vi "Append Front Panel Image.vi"(0 "PDF Report IN":T24(xcontrol), 1 "Scale (%)":sgl=100.0, 3 "Border":T1={"Show?"=FALSE, "Thickness (point)"=0.5, "Color"=0}, 5 "VI reference":refnum<vi>, 9 "visible area only? (T)":bool=TRUE, 11 "error in (no error)":errorcluster, 12 "Caption":string, 14 "Position and indentation":T2={"Alignment"=enum."Center", "X "=0.0, "Y"=0.0, "Indentation"=0.0}) -> (4 "PDF Report OUT":T24(xcontrol), 15 "error out":errorcluster)   [LabVIEW 2012]
doc: "Creates an image of the front panel of the VI you specify in <B>VI reference</B> and appends it to a PDF report.\n\n<B>FRANÇAIS</B>\nCréation de l'image du panneau avant spécifié par <B>VI reference</B> et ajout au rapport PDF.\n\nVersion 1.0\nDeveloped by Jean-Marc Simard\nCopyright © 2010, Exaprom Inc.\nAll rights reserved.\nLicense: BSD\n\nWith iTextSharp 4.1.6 (http://itextsharp.sourceforge.net)\nunder Mozilla Public License Version 1.1\n(http://www.mozilla.org/MPL/MPL-1.1.html)"
uses:
  C:/Users/MaxCorp/Documents/GitHub/TopView/DLL/itextsharp.dll
  GitHub/TopView/DLL/itextsharp.dll
  Controls/Image aligment.ctl
  Controls/Image border.ctl
  Controls/PDF Report Xcontrol/PDF Report.xctl
  Controls/Image alignment and position.ctl
panel:
  out "Size (points)":cluster{"TotalHeight":sgl, "TotalWidth":sgl}
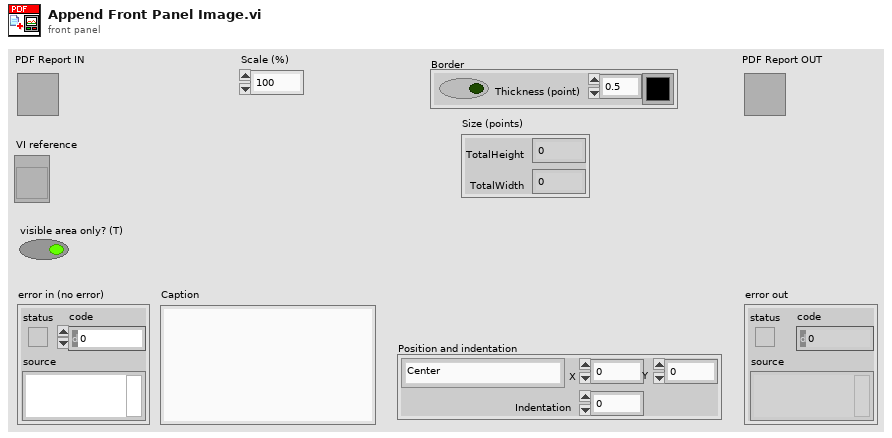
[diagram p1: front panel]
types:
  T1 = typedef "Image border.ctl" = cluster{"Show?":bool, "Thickness (point)":sgl, "Color":u32}
  T2 = typedef "Image alignment and position.ctl" = cluster{"Alignment":T3, "X ":sgl, "Y":sgl, "Indentation":sgl}
  T3 = typedef "Image aligment.ctl" = enum16{"Absolute (X,Y) in mm", "Left", "Center", "Right", "Left (textwrap)", "Right (textwrap)"}
  T4 = typedef "Font cluster.ctl" = cluster{"Name":string, "Size":T5, "Color":T6, "Style":cluster{"Bold":bool, "Italic":bool, "Underline":bool, "Strikeout":bool}}
  T5 = typedef "Font size.ctl" = sgl
  T6 = typedef "Font color.ctl" = u32
  T7 = typedef "Unit.ctl" = enum16{"inch", "mm"}
  T8 = typedef "Paragraphe cluster.ctl" = cluster{" Aligment":T9, "Line spacing":T10}
  T9 = typedef "Texte alignement.ctl" = enum16{"Select", "CENTER", "JUSTIFY", "LEFT", "RIGHT"}
  T10 = typedef "Line spacing.ctl" = enum16{"Select", "1.0", "1.5", "2.0"}
  T11 = typedef "Page dimensions.ctl" = cluster{"Start at page":i32, "Orientation":T12, "widht":sgl, "height":sgl, "Margin left":sgl, "Margin right":sgl, "Margin top":sgl, "Margin bottom":sgl}
  T12 = typedef "Page Orientation.ctl" = enum16{"Portrait", "Landscape"}
  T13 = typedef "Image or Table Caption.ctl" = cluster{"Caption":string, "Separator":string, "Position":enum16{"Above", "Below"}}
  T14 = typedef "Header Footer [ ].ctl" = T15[]
  T15 = typedef "Header Footer cluster.ctl" = cluster{"Start page":i32, "Type":T16, "Alignment":T17, "Vertical Alignement":T18, "Image (%)":sgl, "Page #":T19, "Text":string, "Path":string, "Font":T4, "Font refnum":refnum<k24>, "Line":cluster{"Line":T20, "Thickness (points)":sgl, "Colour":T6}}
  T16 = typedef "Header Footer Type.ctl" = enum16{"Select", "Text", "Text + hyperlink", "Page number", "Image", "Image + hyperlink"}
  T17 = typedef "Header footer horiz alignment.ctl" = enum16{"Left", "Center", "Right"}
  T18 = typedef "Cell Vertical alignment.ctl" = enum16{"TOP", "MIDDLE", "BOTTOM"}
  T19 = typedef "Page number.ctl" = cluster{"Text 1":string, "Text 2":string, "Text 3":string}
  T20 = typedef "Header Footer Line.ctl" = enum16{"No line", "Horizontal line"}
  T21 = typedef "Watermark cluster2.ctl" = cluster{"Show? (F)":bool, "Type":enum16{"Image", "Text"}, "Opacity (%)":sgl, "Rotate(°)":sgl, "Position":cluster{"Position":T22, "X":sgl, "Y":sgl}, "Image path":path, "Scaled(%)":sgl, "Image refnum":refnum<k24>, "Text":string, "Font":cluster{"Name":string, "Size":T5, "Color":T6}, "Font refnum":refnum<k24>, "Alignment":T17, "Automatic":bool}
  T22 = typedef "Watermark Position.ctl" = enum16{"Absolute", "Center (page)", "Center (text section)"}
  T23 = typedef "System Fonts.ctl" = cluster{"Font name [ ]":string[], "Font and file names [ ]":cluster{"Font name":string, "File name":string}[]}
  T24 = cluster{"Document":refnum<k24>, "Writer":refnum<k24>, "Default Font":refnum<k24>, "Default Font cluster":T4, "Path":path, "Unit (default = mm)":T7, "Paragraphe cluster":T8, "Pages dimensions [ ]":T11[], "Captions":cluster{"Image":T13, "Image counter":u16, "Table":T13, "Table counter":u16, "Font":T4}, "Header":T14, "Footer":T14, "Watermark ":T21, "Actual VI name":string, "System Fonts":T23}
  T25 = typedef "imagedata.ctl" = cluster{"image type":i32, "image depth":i32, "image":u8[], "mask":u8[], "colors":u32[], "Rectangle":cluster{"left":i16, "top":i16, "right":i16, "bottom":i16}}
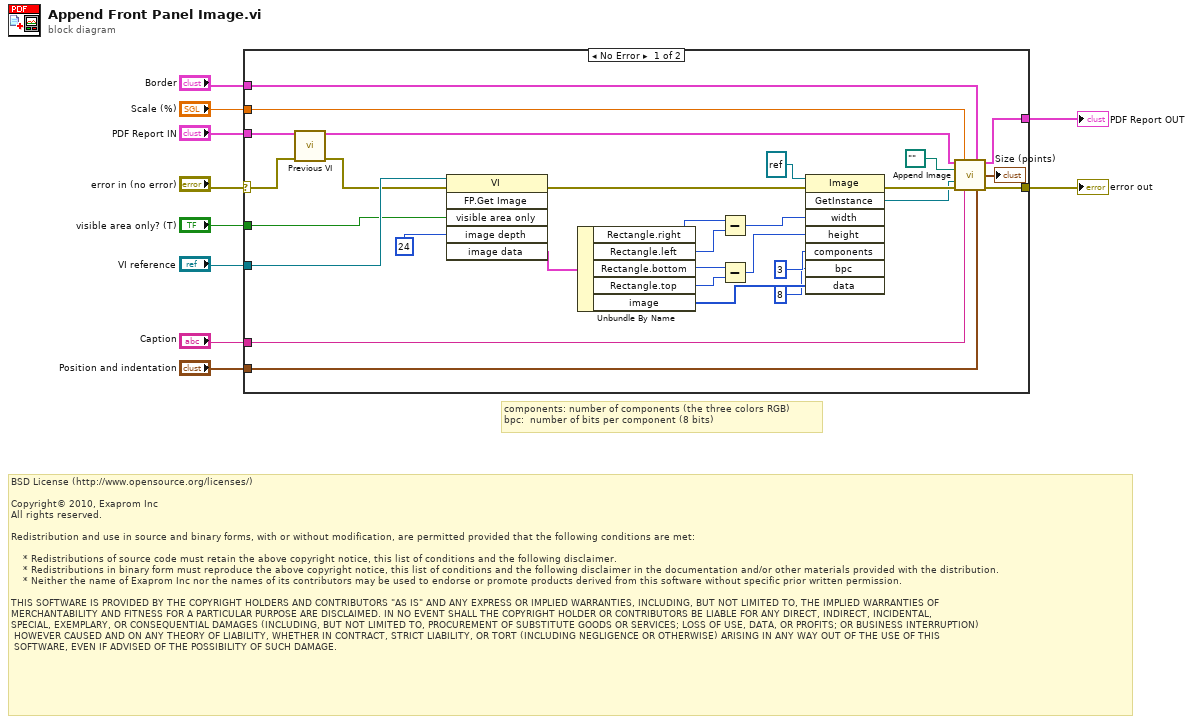
[diagram p0: block diagram]
diagram:
  # "components: number of components (the three colors RGB)\nbpc:  number of bits per component (8 bits)"
  # "BSD License (http://www.opensource.org/licenses/)\n\nCopyright© 2010, Exaprom Inc\nAll rights reserved.\n\nRedistribution and use in source and binary forms, with or without modification, are permitted provided that the following conditions are met:\n\n    * Redistributions of source code must retain the above copyright notice, this list of conditions and the following disclaimer.\n    * Redistributions in binary form must reproduce the above copyright notice, this list of conditions and the following disclaimer in the documentation and/or other materials provided with the distribution.\n    * Neither the name of Exaprom Inc nor the names of its contributors may be used to endorse or promote products derived from this software without specific prior written permission.\n\nTHIS SOFTWARE IS PROVIDED BY THE COPYRIGHT HOLDERS AND CONTRIBUTORS \"AS IS\" AND ANY EXPRESS OR IMPLIED WARRANTIES, INCLUDING, BUT NOT LIMITED TO, THE IMPLIED WARRANTIES OF \nMERCHANTABILITY AND FITNESS FOR A PARTICULAR PURPOSE ARE DISCLAIMED. IN NO EVENT SHALL THE COPYRIGHT HOLDER OR CONTRIBUTORS BE LIABLE FOR ANY DIRECT, INDIRECT, INCIDENTAL,\nSPECIAL, EXEMPLARY, OR CONSEQUENTIAL DAMAGES (INCLUDING, BUT NOT LIMITED TO, PROCUREMENT OF SUBSTITUTE GOODS OR SERVICES; LOSS OF USE, DATA, OR PROFITS; OR BUSINESS INTERRUPTION)\n HOWEVER CAUSED AND ON ANY THEORY OF LIABILITY, WHETHER IN CONTRACT, STRICT LIABILITY, OR TORT (INCLUDING NEGLIGENCE OR OTHERWISE) ARISING IN ANY WAY OUT OF THE USE OF THIS\n SOFTWARE, EVEN IF ADVISED OF THE POSSIBILITY OF SUCH DAMAGE."
  n1 = case shown="No Error" "error in (no error)" {
    selector: "error in (no error)" -> [w12 w41]
    tunnel: [w22 w41] -> w2
    tunnel: "VI reference" -> [w38 _]
    tunnel: [w34 w40] -> w1
    tunnel: "PDF Report IN" -> [w35 w40]
    tunnel: "Caption" -> [w21 _]
    tunnel: "Position and indentation" -> [w20 _]
    tunnel: "Border" -> [w19 _]
    tunnel: "Scale (%)" -> [w18 _]
    tunnel: "visible area only? (T)" -> [w16 _]
    frame No Error {
      n2 = call "Previous VI.vi"("PDF Report IN"=w35, "error in (no error)"=w12) -> ("PDF Report OUT"=w13:T24, "error out"=w11:errorcluster)  [unwired: 12 out]
      n3 = invoke class="VI" method="FP.Get Image"(reference=w38, error in=w11, "visible area only"=w16, "image depth"=24 ("Image Depth")) -> (error out=w39:errorcluster, "image data"=w33:T25)  [unwired: 2 in, 4 out]
      n4 = Unbundle By Name(w33) -> ("Rectangle.right"=w31:i16, "Rectangle.left"=w30:i16, "Rectangle.bottom"=w28:i16, "Rectangle.top"=w27:i16, "image"=w24:u8[])
      n5 = Subtract(x=w31, y=w30) -> (x-y=w29:i16)
      n6 = Subtract(x=w28, y=w27) -> (x-y=w26:i16)
      n7 = invoke class="Image" method="GetInstance"(reference=refnum<k24> refnum ("image"), error in=w39, "width"=w29, "height"=w26, "components"=3, "bpc"=8, "data"=w24) -> (error out=w36:errorcluster, "GetInstance"=w15:refnum<k24>)  [unwired: 1 in, 6 out]
      n8 = call "Append Image.vi"("PDF Report IN"=w13, "Scale (%)"=w18, "Border"=w19, "Image path"=path "" ("path"), "Image Ref iTexSharp"=w15, "error in (no error)"=w36, "Caption"=w21, "Position and indentation"=w20) -> ("PDF Report OUT"=w34:T24, "Size (points)"=→"Size (points)":cluster{"TotalHeight":sgl, "TotalWidth":sgl}, "error out"=w22:errorcluster)  [unwired: 5 out]
    }
    frame Error {
    }
  }
  "error out" <- w2
  "PDF Report OUT" <- w1
